vi "main.vi"() -> ()   [LabVIEW 2020]
uses:
  08f8b78b-8158-40c7-9f7c-aaeb5c1c6287.vi
  <instrlib>/niUSRP/niUSRP Write Tx Data (CDB Cluster).vi
panel:
  out "x << y":i8[](array[numeric])
  out "data 16b":i16[](array[numeric])
  out "check_file":u32
  out "dll end?":bool
  in  "STOP":bool
  out "return type":i8
  in  "START":bool
  out "IQ_arr":i16[](array[numeric])
  in  "CSV/TXT file":path
  in  "height":string="100"
  in  "longtitude":string="138.996902"
  in  "latitude":string="36.318462"
  in  "bin_file_name":string="gps_sim"
  in  "Frequency Offset":dbl=2000000000.0 format="%#_6p"
  out "error out":errorcluster
  in  "Enabled Channel":string(combo)="0"
  out "Coerced Gain":dbl=9.999999999999996 format="%#_6f"
  in  "Device Name":refnum<k15>="192.168.10.2"
  in  "Active Antenna":string="TX1"
  in  "Stop":bool
  in  "Timeout":dbl=10.0
  out "Coerced Carrier Frequency":dbl=2000000000.0 format="%#_6p"
  out "Coerced IQ Rate":dbl=1000000.0 format="%#_6p"
  in  "Gain":dbl=10.0 format="%#_6f"
  in  "Carrier Frequency":dbl=2000000000.0 format="%#_6p"
  in  "IQ Rate":dbl=1000000.0 format="%#_6p"
  in  "Dynamic/RT":bool
  in  "stop":bool
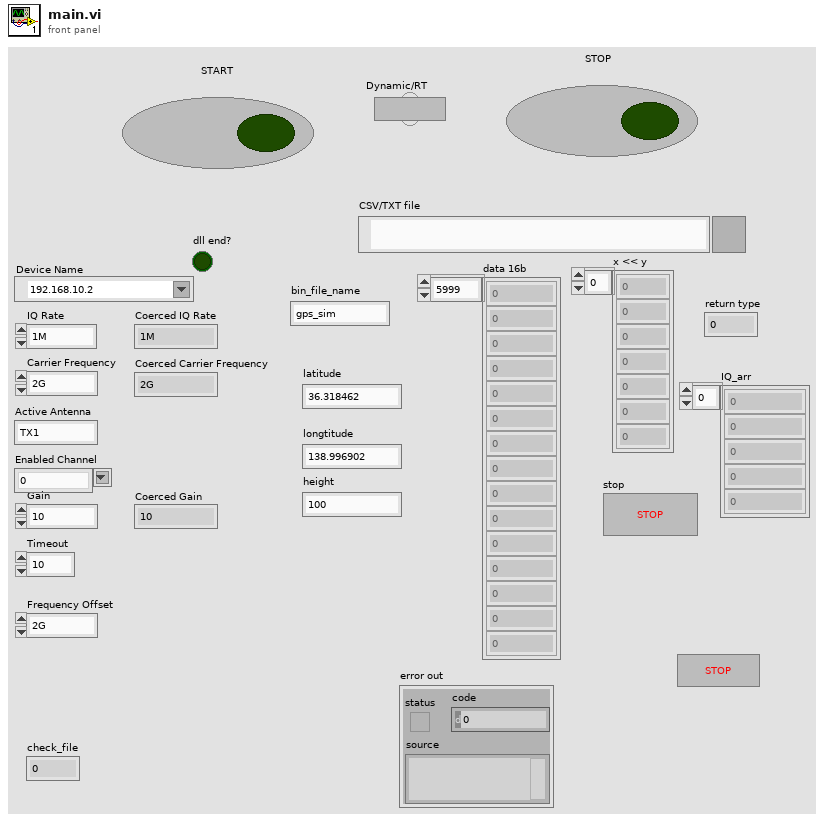
[diagram p1: front panel]
types:
  T1 = enum16{"open", "replace", "create", "open or create", "replace or create", "replace or create with confirmation"}
  T2 = enum16{"big-endian, network order", "native, host order", "little-endian"}
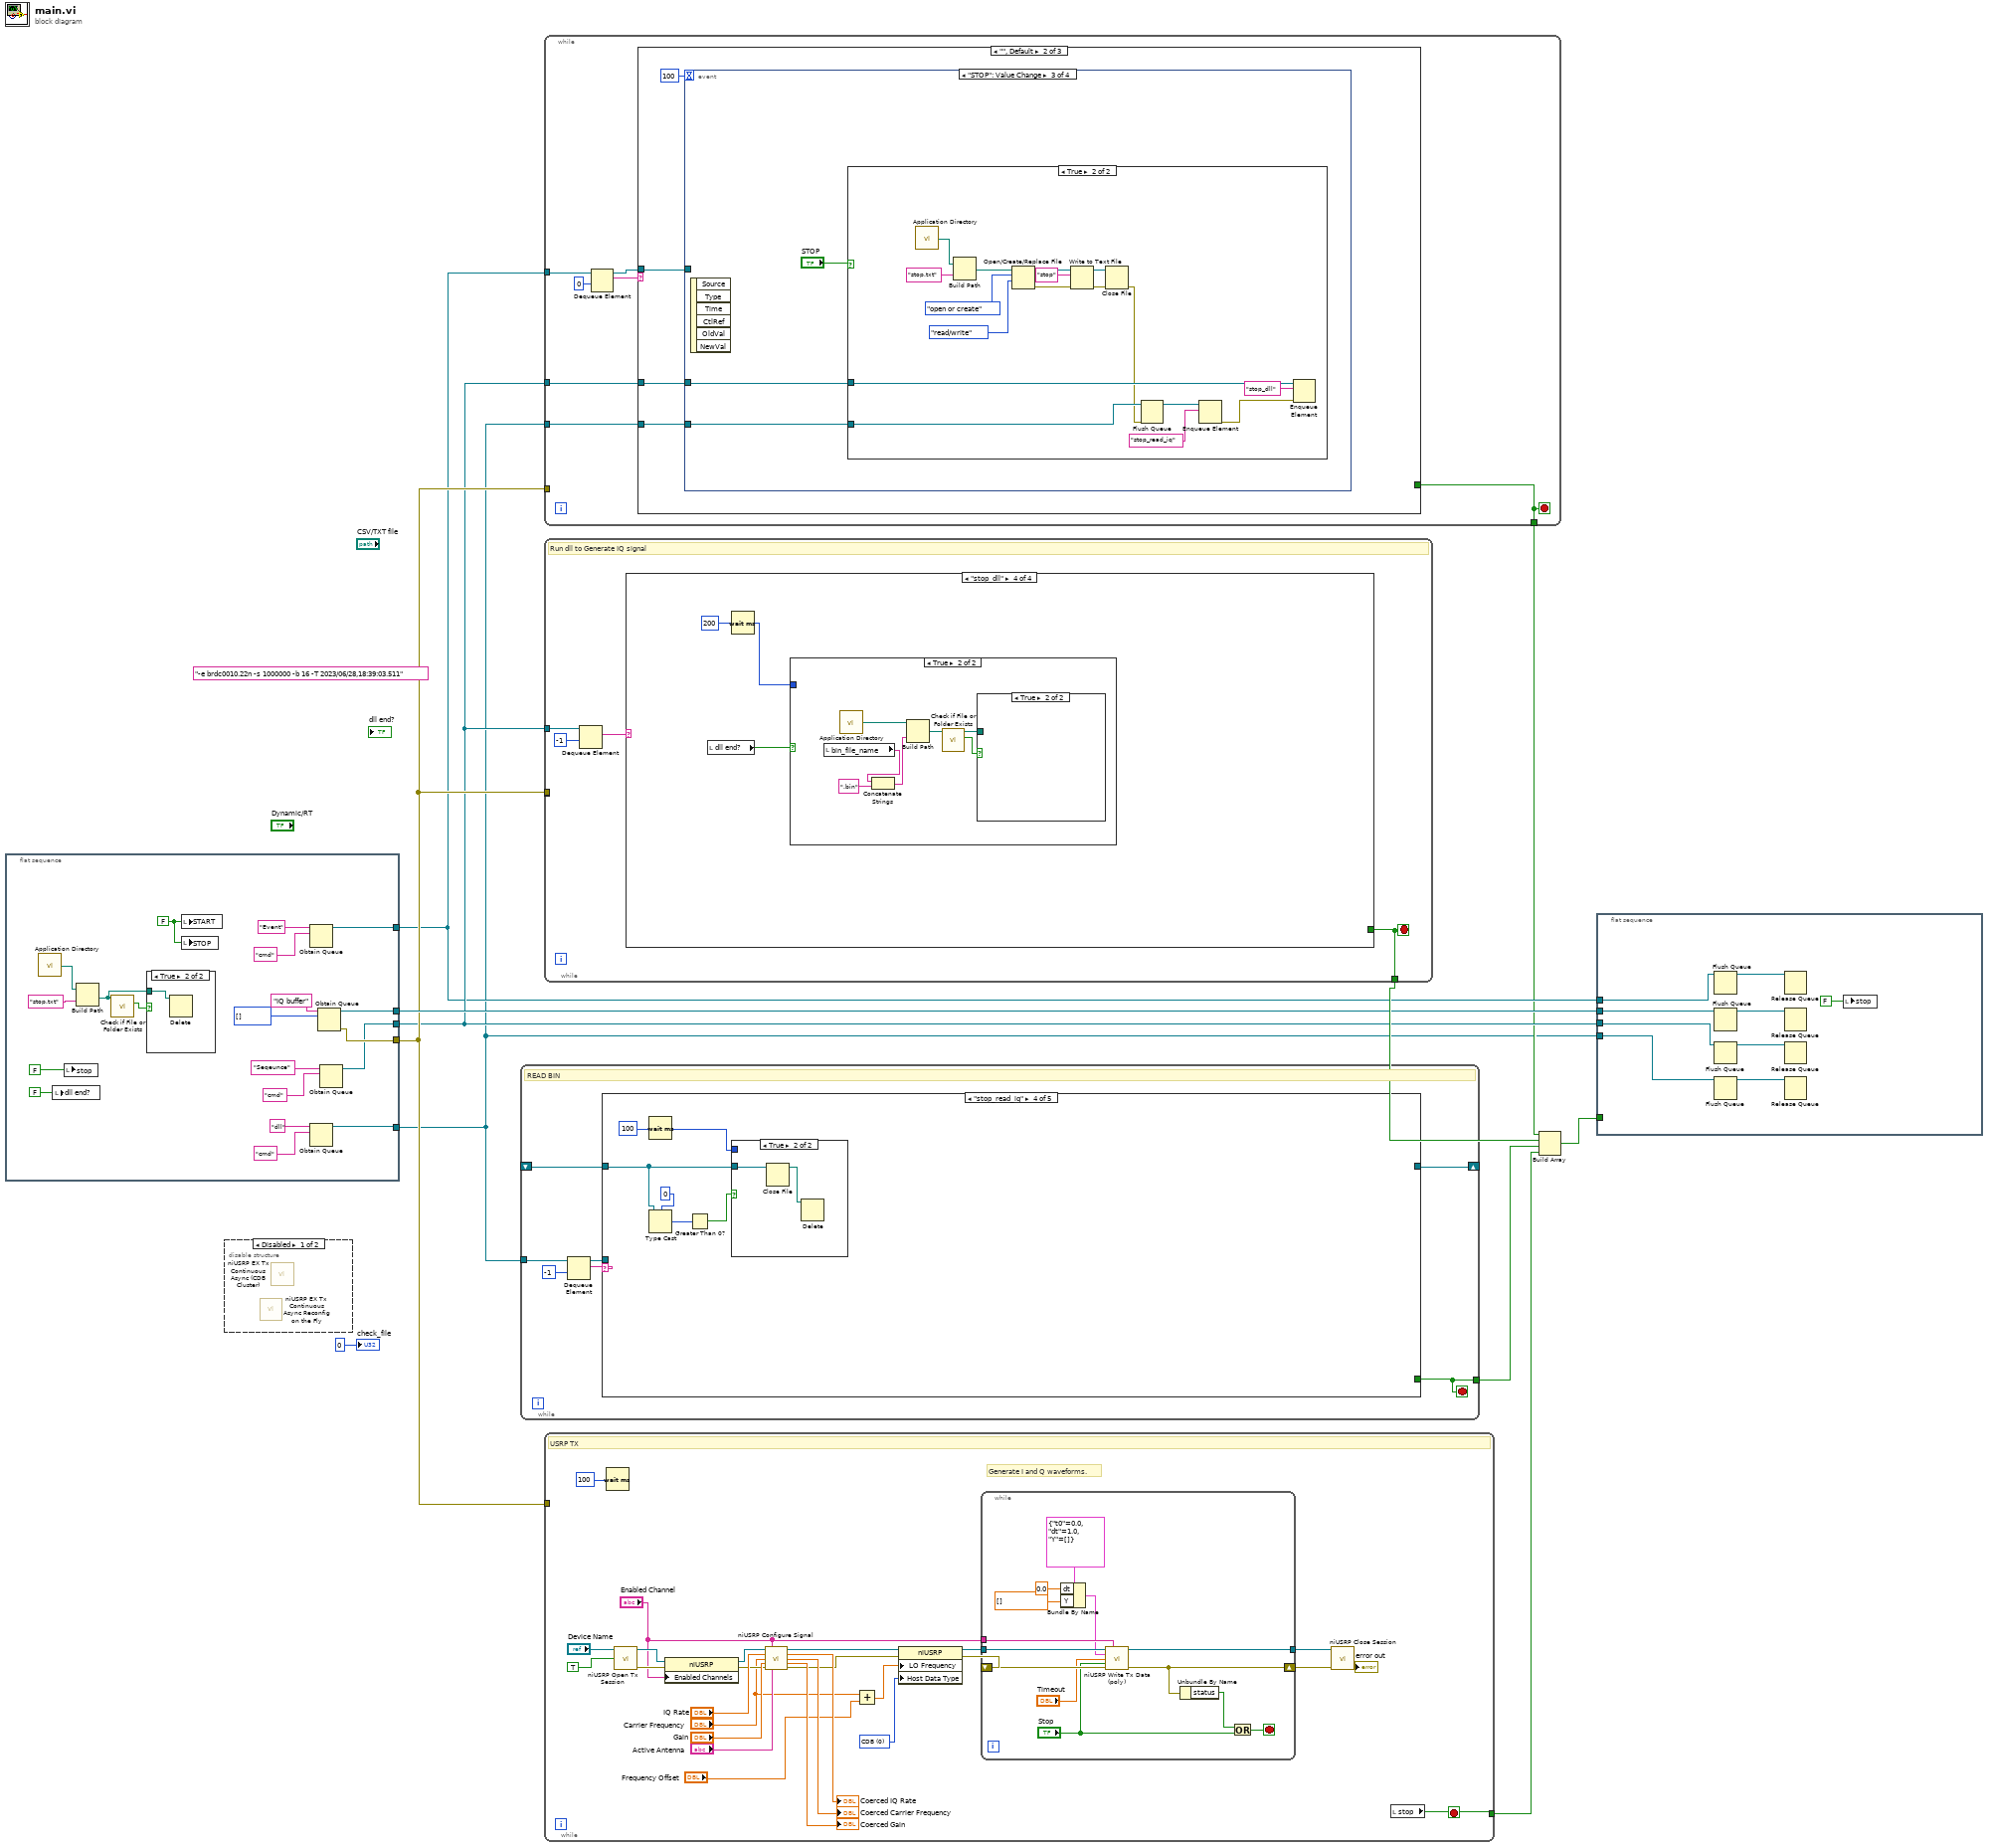
[diagram p0: block diagram]
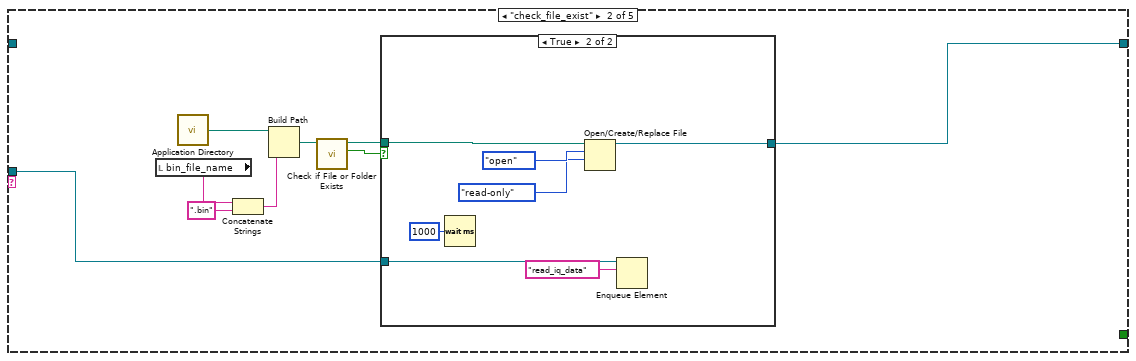
[diagram p3: hidden frame]
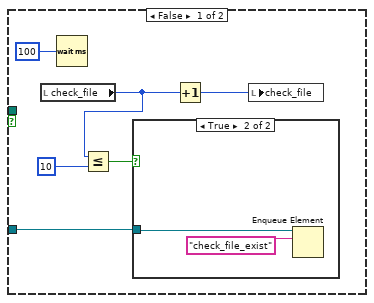
[diagram p4: hidden frame]
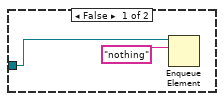
[diagram p5: hidden frame]
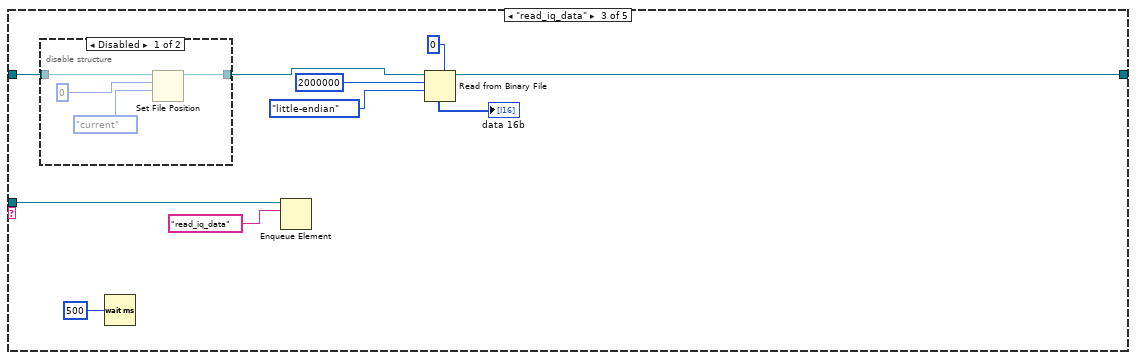
[diagram p6: hidden frame]
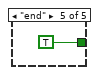
[diagram p9: hidden frame]
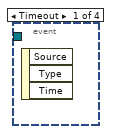
[diagram p11: hidden frame]
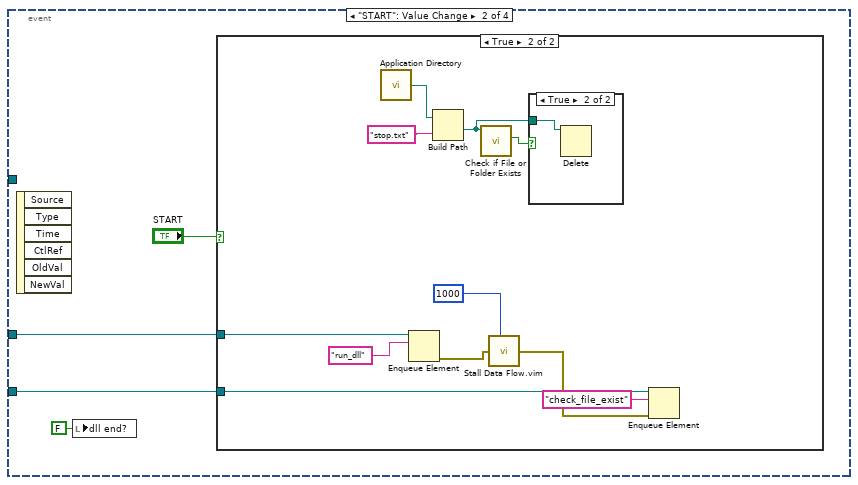
[diagram p12: hidden frame]
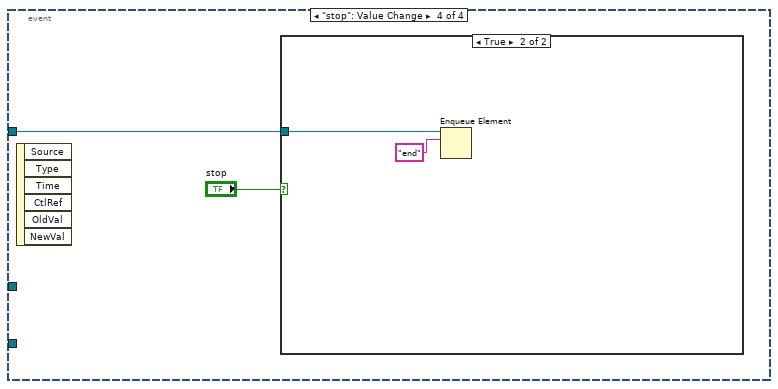
[diagram p16: hidden frame]
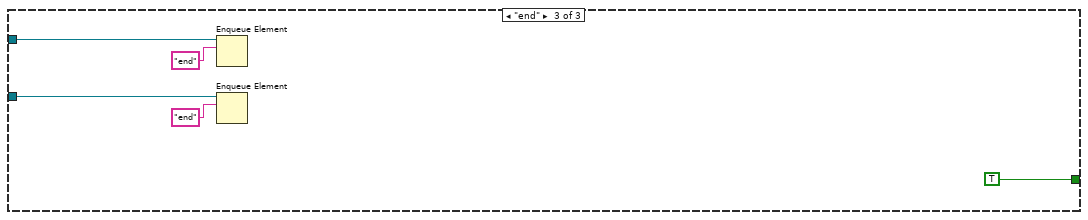
[diagram p18: hidden frame]
diagram:
  (unwired) "-e brdc0010.22n -s 1000000 -b 16 -T 2023/06/28,18:39:03.511" ("param")
  n1 = flat-sequence {
    tunnel: [w30] -> w9
    tunnel: [w29] -> w8
    tunnel: [w20] -> w7
    tunnel: [w17] -> w6
    tunnel: [w14] -> w2
    frame #0 {
      w26 = FALSE ("START")
      n2 = call <vilib>:"Application Directory.vi"() -> ("Application Directory"=w24:path)
      n3 = local write "dll end?"(FALSE ("dll end?")) -> ()
      n4 = local write "stop"(FALSE ("stop")) -> ()
      n5 = Build Path(base path=w24, name or relative path="stop.txt") -> (appended path=w12:path)
      n6 = call <vilib>:"Check if File or Folder Exists.vi"("path"=w12) -> ("file or folder exists?"=w13:bool)  [unwired: 8 in, 2 out]
      n7 = case shown="True" w13 {
        tunnel: w12 -> [_ w32]
        frame False {
        }
        frame True {
          n8 = Delete(path (use dialog)=w32) -> ()  [unwired: 4 in, 3 out]
        }
      }
      n9 = local write "START"(w26) -> ()
      n10 = local write "STOP"(w26) -> ()
      n11 = Obtain Queue(name (unnamed)="Event", element data type="cmd") -> (queue out=w17:refnum<queue>)  [unwired: 3 in, 2 out]
      n12 = Obtain Queue(name (unnamed)="dll", element data type="cmd") -> (queue out=w14:refnum<queue>)  [unwired: 3 in, 2 out]
      n13 = Obtain Queue(name (unnamed)="IQ buffer", element data type=i16[] []) -> (queue out=w30:refnum<queue>, error out=w29:errorcluster)  [unwired: 3 in, 1 out]
      n14 = Obtain Queue(name (unnamed)="Seqeunce", element data type="cmd") -> (queue out=w20:refnum<queue>)  [unwired: 3 in, 2 out]
    }
  }
  n15 = disable-structure shown="Disabled" {
    frame Disabled {
      n16 = call "niUSRP EX Tx Continuous Async Reconfig on the Fly.vi"() -> ()  [unwired: 1 in]
      n17 = call "niUSRP EX Tx Continuous Async (CDB Cluster).vi"() -> ()  [unwired: 1 in]
    }
    frame Enabled {
    }
  }
  n18 = while {
    tunnel: w2 -> [w38]
    tunnel: [w36] -> w3
    shift-right: [w35] -> _
    shift-left: _ -> [w33]
    stop <- w36 stop-if-true
    # "READ BIN"
    n19 = Dequeue Element(queue=w38, timeout in ms (-1)=-1) -> (queue out=w34:refnum<queue>, element=w37:string)  [unwired: 1 in, 2 out]
    n20 = case shown="\"stop_read_iq\"" w37 {
      tunnel: [_ _ _ _ TRUE] -> w36
      tunnel: [_ w44 w70 _ _] -> w35
      tunnel: w34 -> [_ w43 w74 _ _]
      tunnel: w33 -> [_ _ w67 w86 _]
      frame "False", Default {
      }
      frame "check_file_exist" {
        n21 = local read "bin_file_name"() -> (w42:string)
        n22 = call <vilib>:"Application Directory.vi"() -> ("Application Directory"=w48:path)
        n23 = Concatenate Strings(w42, ".bin" ("string")) -> (w41:string)
        n24 = Build Path(base path=w48, name or relative path=w41) -> (appended path=w47:path)
        n25 = call <vilib>:"Check if File or Folder Exists.vi"("path"=w47) -> ("file or folder exists?"=w46:bool, "dup path"=w45:path)  [unwired: 8 in, 1 out]
        n26 = case shown="True" w46 {
          tunnel: w45 -> [_ w65]
          tunnel: [_ w62] -> w44
          tunnel: w43 -> [w50 w60]
          frame False {
            n27 = local read "check_file"() -> (w52:u32)
            n28 = Wait (ms)(milliseconds to wait=u32 100) -> ()  [unwired: 1 out]
            n29 = Less Or Equal?(x=w52, y=u32 10) -> (x <= y?=w49:bool)
            n30 = case shown="True" w49 {
              tunnel: w50 -> [w55 w58]
              frame False {
                n31 = Enqueue Element(queue=w55, element="nothing") -> ()  [unwired: 2 in, 3 out]
              }
              frame True {
                n32 = Enqueue Element(queue=w58, element="check_file_exist") -> ()  [unwired: 2 in, 3 out]
              }
            }
            n33 = Increment(x=w52) -> (x+1=w53:u32)
            n34 = local write "check_file"(w53) -> ()
          }
          frame True {
            n35 = Wait (ms)(milliseconds to wait=u32 1000) -> ()  [unwired: 1 out]
            n36 = Open/Create/Replace File(file path (use dialog)=w65, operation (0:open)=T1."open", access (0:read/write)=enum16{"read/write", "read-only", "write-only"}."read-only") -> (refnum out=w62:refnum<file>)  [unwired: 3 in, 2 out]
            n37 = Enqueue Element(queue=w60, element="read_iq_data") -> ()  [unwired: 2 in, 3 out]
          }
        }
      }
      frame "read_iq_data" {
        n38 = disable-structure shown="Disabled" {
          disable-tunnel: w67 -> [w79 w80]
          disable-tunnel: [w78 w80] -> w66
          frame Disabled {
            n39 = Set File Position(offset (in bytes) (0)=i64 0, refnum=w79, from (0:start)=enum16{"start", "end", "current"}."current") -> (refnum out=w78:refnum<file>)  [unwired: 1 in, 1 out]
          }
          frame Enabled {
          }
        }
        n40 = Wait (ms)(milliseconds to wait=u32 500) -> ()  [unwired: 1 out]
        n41 = Enqueue Element(queue=w74, element="read_iq_data") -> ()  [unwired: 2 in, 3 out]
        n42 = Read from Binary File(5:i16 0, 9:T2."little-endian" ("byte order (0:big-endian, network order)"), 10:2000000 ("count (1)"), 11:w66) -> (2:→"data 16b":i16[], 3:w70:refnum<file>)  [unwired: 2 in, 2 out]
      }
      frame "stop_read_iq" {
        n43 = Wait (ms)(milliseconds to wait=u32 100) -> (millisecond timer value=w81:u32)
        n44 = Type Cast(type=0, x=w86) -> (*(type *) &x=w85:i32)
        n45 = Greater Than 0?(x=w85) -> (x > 0?=w83:bool)
        n46 = case shown="True" w83 {
          tunnel: w86 -> [_ w88]
          tunnel: w81 -> [_ _]
          frame False {
          }
          frame True {
            n47 = Close File(refnum=w88) -> (path=w87:path)  [unwired: 1 in, 1 out]
            n48 = Delete(path (use dialog)=w87) -> ()  [unwired: 4 in, 3 out]
          }
        }
      }
      frame "end" {
      }
    }
  }
  n49 = while {
    tunnel: w8 -> [_]
    tunnel: w6 -> [w96]
    tunnel: w7 -> [w93]
    tunnel: [w91] -> w5
    tunnel: w2 -> [w90]
    stop <- w91 stop-if-true
    n50 = Dequeue Element(queue=w96, timeout in ms (-1)=0) -> (queue out=w92:refnum<queue>, element=w94:string)  [unwired: 1 in, 2 out]
    n51 = case shown="\"\", Default" w94 {
      tunnel: w93 -> [_ w99 w143]
      tunnel: [_ _ TRUE] -> w91
      tunnel: w92 -> [_ w98 _]
      tunnel: w90 -> [_ w97 w141]
      frame "False" {
      }
      frame "", Default {
        n52 = event shown="[2] \"STOP\": Value Change" {
          selector: _ -> [_ _ _ _]
          dyn-events: _ -> [_ _ _ _]
          timeout: 100 -> [_ _ _ _]
          tunnel: w99 -> [_ w102 w118 _]
          tunnel: w98 -> [_ _ _ w137]
          tunnel: w97 -> [_ w101 w117 _]
          event Timeout {
            n53 = event-data() -> ()  [unwired: 1 in, 3 out]
          }
          event "START": Value Change {
            n54 = event-data() -> ()  [unwired: 1 in, 6 out]
            n55 = local write "dll end?"(FALSE ("dll end?")) -> ()
            n56 = case shown="True" "START" {
              tunnel: w102 -> [_ w115]
              tunnel: w101 -> [_ w106]
              frame False {
              }
              frame True {
                n57 = call <vilib>:"Application Directory.vi"() -> ("Application Directory"=w113:path)
                n58 = Enqueue Element(queue=w115, element="run_dll") -> (error out=w109:errorcluster)  [unwired: 2 in, 2 out]
                n59 = Build Path(base path=w113, name or relative path="stop.txt") -> (appended path=w110:path)
                n60 = call <vilib>:"Check if File or Folder Exists.vi"("path"=w110) -> ("file or folder exists?"=w111:bool)  [unwired: 8 in, 2 out]
                n61 = call "Stall Data Flow.vim"("value in"=w109, "milliseconds to wait"=u32 1000) -> ("value out"=w107:errorcluster)  [unwired: 1 out]
                n62 = case shown="True" w111 {
                  tunnel: w110 -> [_ w116]
                  frame False {
                  }
                  frame True {
                    n63 = Delete(path (use dialog)=w116) -> ()  [unwired: 4 in, 3 out]
                  }
                }
                n64 = Enqueue Element(queue=w106, element="check_file_exist", error in (no error)=w107) -> ()  [unwired: 1 in, 3 out]
              }
            }
          }
          event "STOP": Value Change {
            n65 = event-data() -> ()  [unwired: 1 in, 6 out]
            n66 = case shown="True" "STOP" {
              tunnel: w118 -> [_ w126]
              tunnel: w117 -> [_ w124]
              frame False {
              }
              frame True {
                n67 = call <vilib>:"Application Directory.vi"() -> ("Application Directory"=w136:path)
                n68 = Build Path(base path=w136, name or relative path="stop.txt") -> (appended path=w134:path)
                n69 = Open/Create/Replace File(file path (use dialog)=w134, operation (0:open)=T1."open or create", access (0:read/write)=enum16{"read/write", "read-only", "write-only"}."read/write") -> (refnum out=w132:refnum<file>, error out=w130:errorcluster)  [unwired: 3 in, 1 out]
                n70 = Write to Text File(file (use dialog)=w132, text="stop", error in=w130) -> (refnum out=w131:refnum<file>, error out=w129:errorcluster)  [unwired: 1 in, 1 out]
                n71 = Close File(refnum=w131, error in=w129) -> (error out=w121:errorcluster)  [unwired: 1 out]
                n72 = Flush Queue(queue=w124, error in (no error)=w121) -> (queue out=w123:refnum<queue>)  [unwired: 2 out]
                n73 = Enqueue Element(queue=w123, element="stop_read_iq") -> (error out=w120:errorcluster)  [unwired: 2 in, 2 out]
                n74 = Enqueue Element(queue=w126, element="stop_dll", error in (no error)=w120) -> ()  [unwired: 1 in, 3 out]
              }
            }
          }
          event "stop": Value Change {
            n75 = event-data() -> ()  [unwired: 1 in, 6 out]
            n76 = case shown="True" "stop" {
              tunnel: w137 -> [_ w139]
              frame False {
              }
              frame True {
                n77 = Enqueue Element(queue=w139, element="end") -> ()  [unwired: 2 in, 3 out]
              }
            }
          }
        }
      }
      frame "end" {
        n78 = Enqueue Element(queue=w143, element="end") -> ()  [unwired: 2 in, 3 out]
        n79 = Enqueue Element(queue=w141, element="end") -> ()  [unwired: 2 in, 3 out]
      }
    }
  }
  n80 = while {
    tunnel: [w146] -> w11
    tunnel: [w150] -> _
    tunnel: w8 -> [w150]
    tunnel: w7 -> [w149]
    stop <- w146 stop-if-true
    # "Run dll to Generate IQ signal"
    n81 = Dequeue Element(queue=w149, timeout in ms (-1)=-1) -> (element=w147:string)  [unwired: 1 in, 3 out]
    n82 = case shown="\"stop_dll\"" w147 {
      tunnel: [_ TRUE _ _] -> w146
      frame "False", Default {
      }
      frame "end" {
      }
      frame "run_dll" {
        w169 = "," ("string")
        n83 = call <vilib>:"Application Directory.vi"() -> ("Application Directory"=w173:path)
        n84 = local read "Dynamic/RT"() -> (w156:bool)
        n85 = Concatenate Strings(" -l " ("string"), "latitude", w169, "longtitude", w169, "height") -> (w164:string)
        n86 = Path To String(path=w173) -> (string=w174:string)
        n87 = Build Path(base path=w173, name or relative path="GPS_SIM_CREATE_BIN.dll") -> (appended path=w175:path)
        n88 = case shown="False" w156 {
          tunnel: ["" ("string") " -r" ("string")] -> w155
          frame False {
          }
          frame True {
          }
        }
        n89 = Concatenate Strings(" -o " ("string"), "bin_file_name") -> (w163:string)
        n90 = Concatenate Strings("-e brdc0010.22n -s 1000000" ("param"), w164, w163, w155) -> (w162:string)
        n91 = Initialize Array(i16 0 ("element"), 200000 ("dimension size")) -> (w159:i16[])
        n92 = dll-call lib="PTH2iabs CUsersduygaOneDriveデスクトップWORKS\nNissan GPS\tbuild dllGPS_SIM_CREATE_BIN.dll" fn="GPS_create_bin"(path in=w175, "param"=w162, "base_path"=w174, "IQ_arr"=w159) -> (error out=w157:errorcluster, "return type"=→"return type":i8, "IQ_arr"=w154:i16[])  [unwired: 4 in, 1 out]
        "IQ_arr" <- w154
        n93 = flat-sequence {
          tunnel: w157 -> [_]
          frame #0 {
            w179 = FALSE ("START")
            n94 = local write "dll end?"(TRUE ("dll end?")) -> ()
            n95 = local write "START"(w179) -> ()
            n96 = local write "STOP"(w179) -> ()
          }
        }
        n97 = Logical Shift(y=i16 -4, x=w154) -> (x << y=→"x << y":i16[])
      }
      frame "stop_dll" {
        n98 = local read "dll end?"() -> (w182:bool)
        n99 = Wait (ms)(milliseconds to wait=u32 200) -> (millisecond timer value=w181:u32)
        n100 = case shown="True" w182 {
          tunnel: w181 -> [_ _]
          frame False {
          }
          frame True {
            n101 = local read "bin_file_name"() -> (w184:string)
            n102 = call <vilib>:"Application Directory.vi"() -> ("Application Directory"=w189:path)
            n103 = Concatenate Strings(w184, ".bin" ("string")) -> (w185:string)
            n104 = Build Path(base path=w189, name or relative path=w185) -> (appended path=w190:path)
            n105 = call <vilib>:"Check if File or Folder Exists.vi"("path"=w190) -> ("file or folder exists?"=w188:bool, "dup path"=w187:path)  [unwired: 8 in, 1 out]
            n106 = case shown="True" w188 {
              tunnel: w187 -> [_ _]
              frame False {
              }
              frame True {
              }
            }
          }
        }
      }
    }
  }
  n107 = while {
    tunnel: [w216] -> w4
    tunnel: w8 -> [_]
    stop <- w216 stop-if-true
    w192 = 0 items=["CDB", "I16"] ("Configuration:Advanced:Host Data Type")
    # "Generate I and Q waveforms."
    # "USRP TX"
    n108 = Wait (ms)(milliseconds to wait=u32 100) -> ()  [unwired: 1 out]
    n109 = call <instrlib>:"niUSRP Open Tx Session.vi"("device names"="Device Name", "reset"=TRUE) -> ("session handle out"=w206:refnum<k15>, "error out"=w205:errorcluster)  [unwired: 12 in]
    n110 = property class="niUSRP"(reference=w206, error in=w205, "Enabled Channels"="Enabled Channel") -> (reference out=w204:refnum<k15>, error out=w203:errorcluster)
    n111 = call <instrlib>:"niUSRP Configure Signal.vi"("session handle"=w204, "channel list"="Enabled Channel", "IQ rate"="IQ Rate", "carrier frequency"="Carrier Frequency", "gain"="Gain", "error in (no error)"=w203, "active antenna"="Active Antenna") -> ("session handle out"=w199:refnum<k15>, "coerced IQ rate"=→"Coerced IQ Rate":dbl, "coerced carrier frequency"=→"Coerced Carrier Frequency":dbl, "coerced gain"=→"Coerced Gain":dbl, "error out"=w194:errorcluster)  [unwired: 4 in]
    n112 = Add(x="Carrier Frequency", y="Frequency Offset") -> (x+y=w195:dbl)
    n113 = property class="niUSRP"(reference=w199, error in=w194, "LO Frequency"=w195, "Host Data Type"=w192) -> (reference out=w198:refnum<k15>, error out=w193:errorcluster)
    n114 = while {
      tunnel: w198 -> [w228]
      tunnel: [w225] -> w213
      shift-right: [w224] -> w212
      shift-left: w193 -> [w227]
      tunnel: "Enabled Channel" -> [w221]
      stop <- w229 stop-if-true
      n115 = Bundle By Name(cluster=cluster{"t0":dbl, "dt":dbl, "Y":cdb[]} {"t0"=0.0, "dt"=1.0, "Y"=[]} ("data"), "dt"=0.0, "Y"=cdb[] []) -> (w219:cluster{"t0":dbl, "dt":dbl, "Y":cdb[]})
      n116 = call-poly <instrlib>:"niUSRP Write Tx Data (poly).vi"("session handle"=w228, "channel list"=w221, "data"=w219, "timeout"="Timeout", "end of data?"="Stop", "error in (no error)"=w227) -> ("session handle out"=w225:refnum<k15>, "error out"=w224:errorcluster)  [unwired: 8 in]
      n117 = Unbundle By Name(w224) -> ("status"=w223:bool)
      n118 = Or(x=w223, y="Stop") -> (x .or. y?=w229:bool)
    }
    n119 = call <instrlib>:"niUSRP Close Session.vi"("session handle"=w213, "error in (no error)"=w212) -> ("error out"=→"error out":errorcluster)  [unwired: 13 in]
    n120 = local read "stop"() -> (w216:bool)
  }
  n121 = Build Array(w5, w11, w3, w4) -> (w10:bool[])
  n122 = flat-sequence {
    tunnel: w10 -> [_]
    tunnel: w9 -> [w237]
    tunnel: w7 -> [w235]
    tunnel: w6 -> [w233]
    tunnel: w2 -> [w230]
    frame #0 {
      n123 = Flush Queue(queue=w233) -> (queue out=w232:refnum<queue>)  [unwired: 1 in, 2 out]
      n124 = Flush Queue(queue=w237) -> (queue out=w238:refnum<queue>)  [unwired: 1 in, 2 out]
      n125 = Flush Queue(queue=w235) -> (queue out=w236:refnum<queue>)  [unwired: 1 in, 2 out]
      n126 = Flush Queue(queue=w230) -> (queue out=w231:refnum<queue>)  [unwired: 1 in, 2 out]
      n127 = Release Queue(queue=w232) -> ()  [unwired: 2 in, 3 out]
      n128 = Release Queue(queue=w238) -> ()  [unwired: 2 in, 3 out]
      n129 = Release Queue(queue=w236) -> ()  [unwired: 2 in, 3 out]
      n130 = Release Queue(queue=w231) -> ()  [unwired: 2 in, 3 out]
      n131 = local write "stop"(FALSE ("stop")) -> ()
    }
  }
  "check_file" <- u32 0 ("check_file")
